vi "Decode Encoder.vi"(0 "RAW Data":u16[](array[numeric])) -> (4 "result":u32)   [LabVIEW 2019, in "MB_ENGINE.lvclass"]
uses:
  MB_ENGINE.lvclass
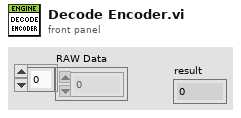
[diagram p1: front panel]
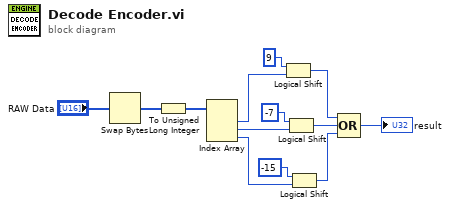
[diagram p0: block diagram]
diagram:
  n1 = Swap Bytes(anything="RAW Data") -> (byte swapped=w12:u16[])
  n2 = To Unsigned Long Integer(number=w12) -> (unsigned 32bit integer=w11:u32[])
  n3 = Index Array(array=w11) -> (element #1=w10:u32, element #2=w6:u32, element #3=w5:u32)  [unwired: 3 in]
  n4 = Logical Shift(y=i16 9, x=w10) -> (x << y=w9:u32)
  n5 = Logical Shift(y=i16 -7, x=w6) -> (x << y=w8:u32)
  n6 = Logical Shift(y=i16 -15, x=w5) -> (x << y=w7:u32)
  n7 = Compound Arithmetic op=OR(w9, w8, w7) -> (→"result":u32)
